vi "Notify.vi"(8 "error in (no error)":errorcluster, 10 "String":string, 11 "Notifier in":refnum<notifier>) -> (0 "error out":errorcluster)   [LabVIEW 2014]
panel:
  # "LICENSED MATERIALS – PROPERTY OF IBM\nCopyright IBM Corp. 2016,\nALL RIGHTS RESERVED"
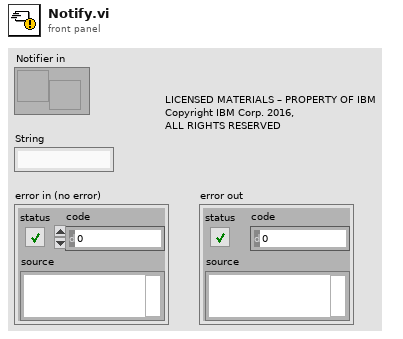
[diagram p1: front panel]
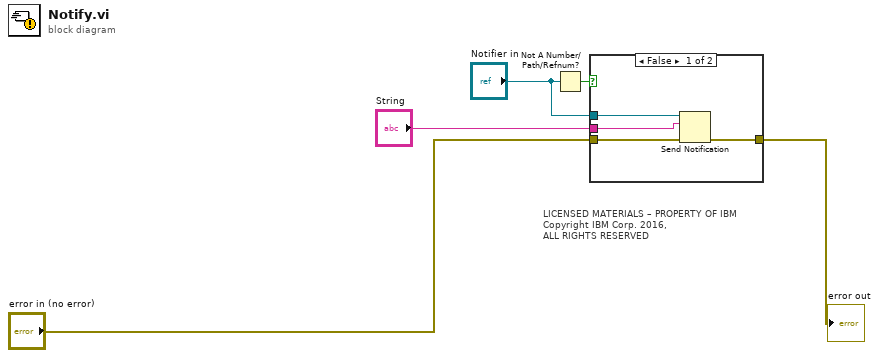
[diagram p0: block diagram]
diagram:
  # "LICENSED MATERIALS – PROPERTY OF IBM\nCopyright IBM Corp. 2016,\nALL RIGHTS RESERVED"
  n1 = Not A Number/Path/Refnum?(number/path/refnum="Notifier in") -> (NaN/Path/Refnum?=w2:bool)
  n2 = case shown="False" w2 {
    tunnel: "error in (no error)" -> [w9 w10]
    tunnel: [w8 w10] -> w1
    tunnel: "Notifier in" -> [w7 _]
    tunnel: "String" -> [w6 _]
    frame False {
      n3 = Send Notification(notification=w6, notifier=w7, error in (no error)=w9) -> (error out=w8:errorcluster)  [unwired: 1 out]
    }
    frame True {
    }
  }
  "error out" <- w1
